vi "平方根（牛顿迭代法）.vi"(1 "a":dbl) -> (0 "sqrt(a)":dbl)   [LabVIEW 2012]
doc: "功能：\n\n求三位数中的水仙花数\n\n水仙花数的定义：\n\n所谓水仙花数，是指一个三位数，其各个位数的立方和等于该数本身，比如：\n\n153=1^3+5^+3^\n\ncsxcs_366创建"
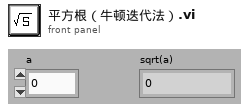
[diagram p1: front panel]
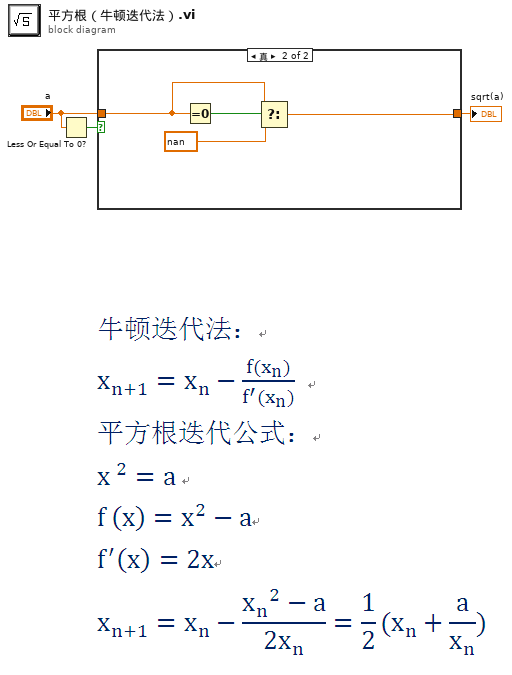
[diagram p0: block diagram]
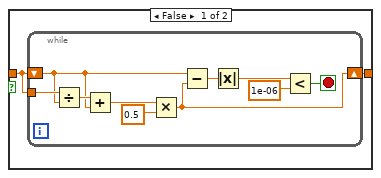
[diagram p2: hidden frame]
diagram:
  n1 = Less Or Equal To 0?(x="a") -> (x <= 0?=w2:bool)
  n2 = case shown="真" w2 {
    tunnel: "a" -> [w5 w18]
    tunnel: [w4 w16] -> w1
    frame False {
      n3 = while {
        tunnel: w5 -> [w15]
        shift-right: [w6] -> w4
        shift-left: w5 -> [w7]
        stop <- w8 stop-if-true
        n4 = Divide(x=w15, y=w7) -> (x/y=w14:dbl)
        n5 = Add(x=w14, y=w7) -> (x+y=w13:dbl)
        n6 = Multiply(x=w13, y=0.5) -> (x*y=w6:dbl)
        n7 = Subtract(x=w7, y=w6) -> (x-y=w11:dbl)
        n8 = Absolute Value(x=w11) -> (abs(x)=w10:dbl)
        n9 = Less?(x=w10, y=1e-06) -> (x < y?=w8:bool)
      }
    }
    frame True {
      n10 = Equal To 0?(x=w18) -> (x = 0?=w19:bool)
      n11 = Select(t=w18, s=w19, f=nan) -> (s? t:f=w16:dbl)
    }
  }
  "sqrt(a)" <- w1
